vi "EncryptWaveform.vi"() -> ()   [LabVIEW 2012]
uses:
  <vilib>/Waveform/WDTFileIO.llb/ Write Waveform to File.vi
  <vilib>/Waveform/WDTFileIO.llb/ Write Waveforms to File (1D).vi
panel:
  out "Message":string
  out "Encrypted":string
  out "Input Sound File":string
  in  "Message Title":string
  out "Encryption":string
  in  "Base Path":path
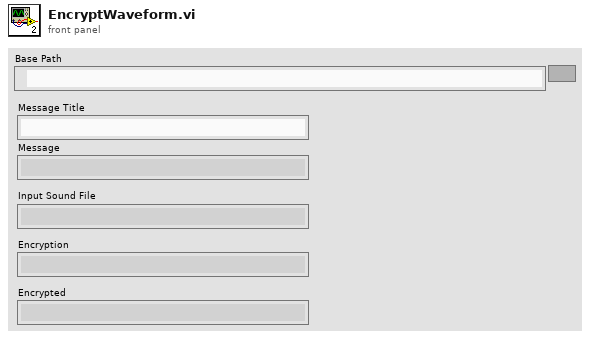
[diagram p1: front panel]
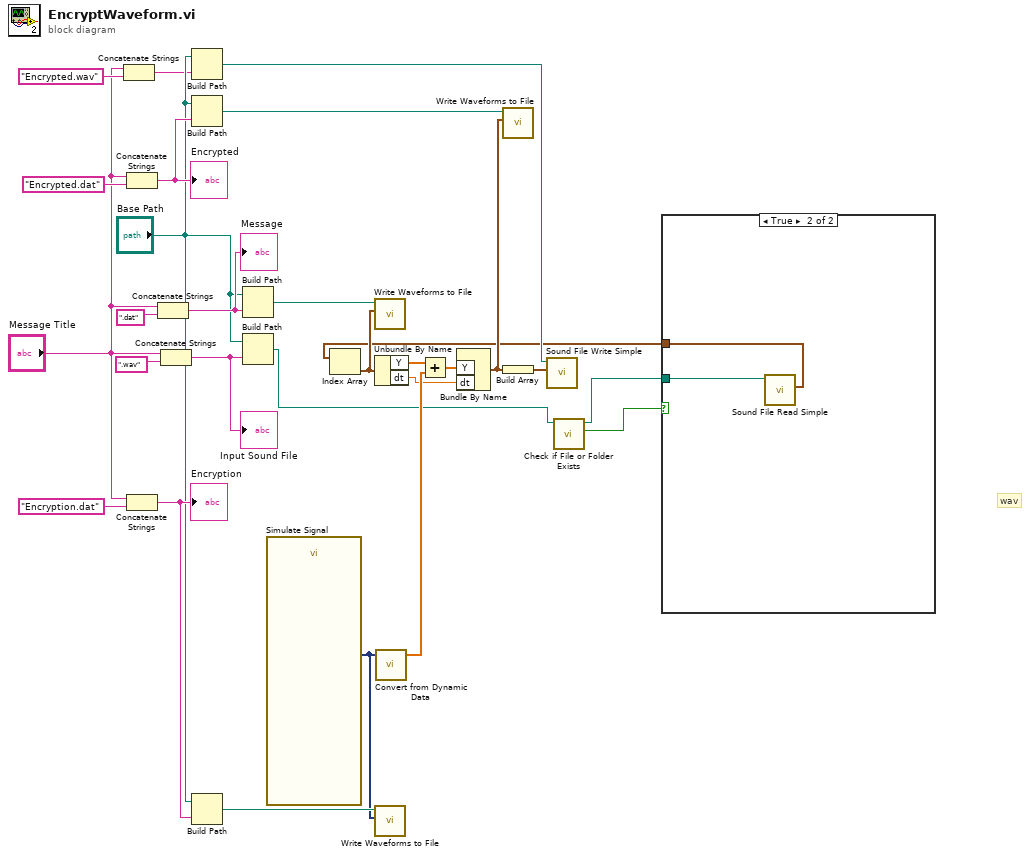
[diagram p0: block diagram]
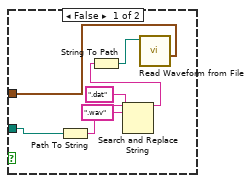
[diagram p2: hidden frame]
diagram:
  # "wav"
  n1 = Concatenate Strings("Message Title", "Encrypted.wav" ("string")) -> (w8:string)
  n2 = Concatenate Strings("Message Title", "Encrypted.dat" ("string")) -> (w17:string)
  "Encrypted" <- w17
  n3 = Concatenate Strings("Message Title", "Encryption.dat" ("string")) -> (w13:string)
  "Encryption" <- w13
  n4 = Concatenate Strings("Message Title", ".dat" ("string")) -> (w12:string)
  "Message" <- w12
  n5 = Concatenate Strings("Message Title", ".wav" ("string")) -> (w15:string)
  "Input Sound File" <- w15
  n6 = Build Path(base path="Base Path", name or relative path=w8) -> (appended path=w7:path)
  n7 = Build Path(base path="Base Path", name or relative path=w17) -> (appended path=w20:path)
  n8 = Build Path(base path="Base Path", name or relative path=w13) -> (appended path=w28:path)
  n9 = Build Path(base path="Base Path", name or relative path=w12) -> (appended path=w27:path)
  n10 = Build Path(base path="Base Path", name or relative path=w15) -> (appended path=w4:path)
  n11 = call "Simulate Signal"() -> ("Sine with Periodic Noise"=w25:dynamicdata)  [unwired: 14 in, 1 out]
  n12 = call-poly <vilib>:"Write Waveforms to File.vi"("waveform array"=w25, "file path (dialog if empty)"=w28) -> ()  [unwired: 8 in, 2 out]
  n13 = call "Convert from Dynamic Data"("Dynamic Data Type"=w25) -> ("Array"=w23:dbl[])  [unwired: 3 in]
  n14 = call <vilib>:"Check if File or Folder Exists.vi"("path"=w4) -> ("file or folder exists?"=w1:bool, "dup path"=w3:path)  [unwired: 8 in, 1 out]
  n15 = case shown="True" w1 {
    tunnel: w3 -> [w35 w37]
    tunnel: [w29 w36] -> w2
    frame False {
      n16 = Path To String(path=w35) -> (string=w34:string)
      n17 = Search and Replace String(input string=w34, search string=".wav", replace string=".dat" ("replace string (\"\")")) -> (result string=w31:string)  [unwired: 5 in, 3 out]
      n18 = String To Path(string=w31) -> (path=w30:path)
      n19 = call <vilib>:"Read Waveform from File.vi"("file path (dialog if empty)"=w30) -> ("all waveforms in record"=w29:waveform(dbl)[])  [unwired: 5 in, 3 out]
    }
    frame True {
      n20 = call <vilib>:"Sound File Read Simple.vi"("path"=w37) -> ("data"=w36:waveform(dbl)[])  [unwired: 7 in, 3 out]
    }
  }
  n21 = Index Array(array=w2) -> (element=w26:waveform(dbl))  [unwired: 1 in]
  n22 = call-poly <vilib>:"Write Waveforms to File.vi"("waveform"=w26, "file path (dialog if empty)"=w27) -> ()  [unwired: 8 in, 2 out]
  n23 = Unbundle By Name(w26) -> ("Y"=w24:dbl[], "dt"=w21:dbl)
  n24 = Add(x=w24, y=w23) -> (x+y=w22:dbl[])
  n25 = Bundle By Name("Y"=w22, "dt"=w21) -> (w5:waveform(dbl))  [unwired: 1 in]
  n26 = call-poly <vilib>:"Write Waveforms to File.vi"("waveform"=w5, "file path (dialog if empty)"=w20) -> ()  [unwired: 8 in, 2 out]
  n27 = Build Array(w5) -> (w6:waveform(dbl)[])
  n28 = call <vilib>:"Sound File Write Simple.vi"("data"=w6, "path"=w7) -> ()  [unwired: 8 in, 2 out]
